vi "Test-Climb.vi"() -> ()   [LabVIEW 2023]
doc: "This VI implements the framework and scheduler for your robotics program. It should not be necessary to modify the framework. You are expected to add your code to the VIs called from Robot Main - the ones located in the Team Code folder within the project."
uses:
  <vilib>/Rock Robotics/WPI/DriverStation/WPI_DriverStationRobotMode2.ctl
  Climb/ClimbStates.ctl
  Robot Global Data.vi
  <vilib>/Rock Robotics/WPI/ThirdParty/JAS_Junk/TrajLib/Trajectory_Library.lvlib
panel:
  out "ClimbStates":T1
  in  "ClimbIncReach":bool
  in  "ClimbIncPull":bool
  in  "ClimbReach":bool
  in  "ClimbPull":bool
  in  "ClimbRest":bool
  out "Wrist Chart":T2(graph)
  out "Battery_Volts":dbl format="%9.1f"
  out "Climbe SP Deg":dbl format="%9.1f"
  out "At Outer Limit":bool
  out "At Inner Limit":bool
  out "Climb Anble Deg":dbl format="%9.1f"
  out "Robot Mode":T3
  out "MotorOutDmd":dbl format="%9.2f"
  in  "error in (no error)":errorcluster
  in  "Finish":bool
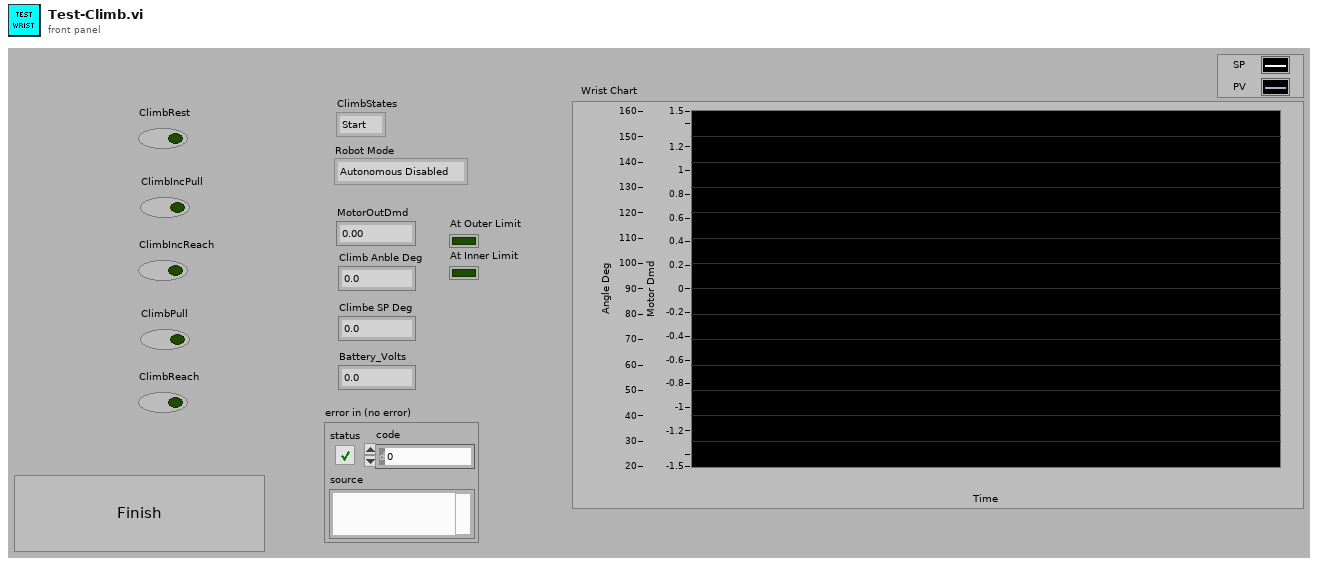
[diagram p1: front panel]
types:
  T1 = typedef "ClimbStates.ctl" = enum16{"Start", "WaitForCommands", "ClimbRest", "ClimbReach", "ClimbPull"}
  T2 = cluster{"ElevatorPosDemandHeight":dbl, "ElevHeightInch":dbl, "MotorDemand":dbl}
  T3 = typedef "WPI_DriverStationRobotMode2.ctl" = enum16{"Autonomous Disabled", "Autonomous Enabled", "Teleop Disabled", "Teleop Enabled", "Disconnected", "Finish", "Test Disabled", "Test Enabled", "Emergency Stopped"}
  T4 = cluster{"WristSP Deg 2":dbl, "ClimbPositionDegrees":dbl, "MotorDemand":dbl}
  T5 = typedef "WPI_DriverStationMatch Info.ctl" = cluster{"Autonomous Elapsed Seconds":dbl, "TeleOp Elapsed Seconds":dbl, "Disabled Elapsed Seconds":dbl, "Visited Autonomous":bool, "Visited TeleOp":bool, "Visited Disabled":bool, "Autonomous Settings":cluster{"Autonomous Style":enum16{"Iterative", "Independent"}, "VI Refnum":refnum<vi>}}
  T6 = typedef "WPI_DriverStationDerivedRobotMode.ctl" = enum16{"Init", "Execute", "Stop"}
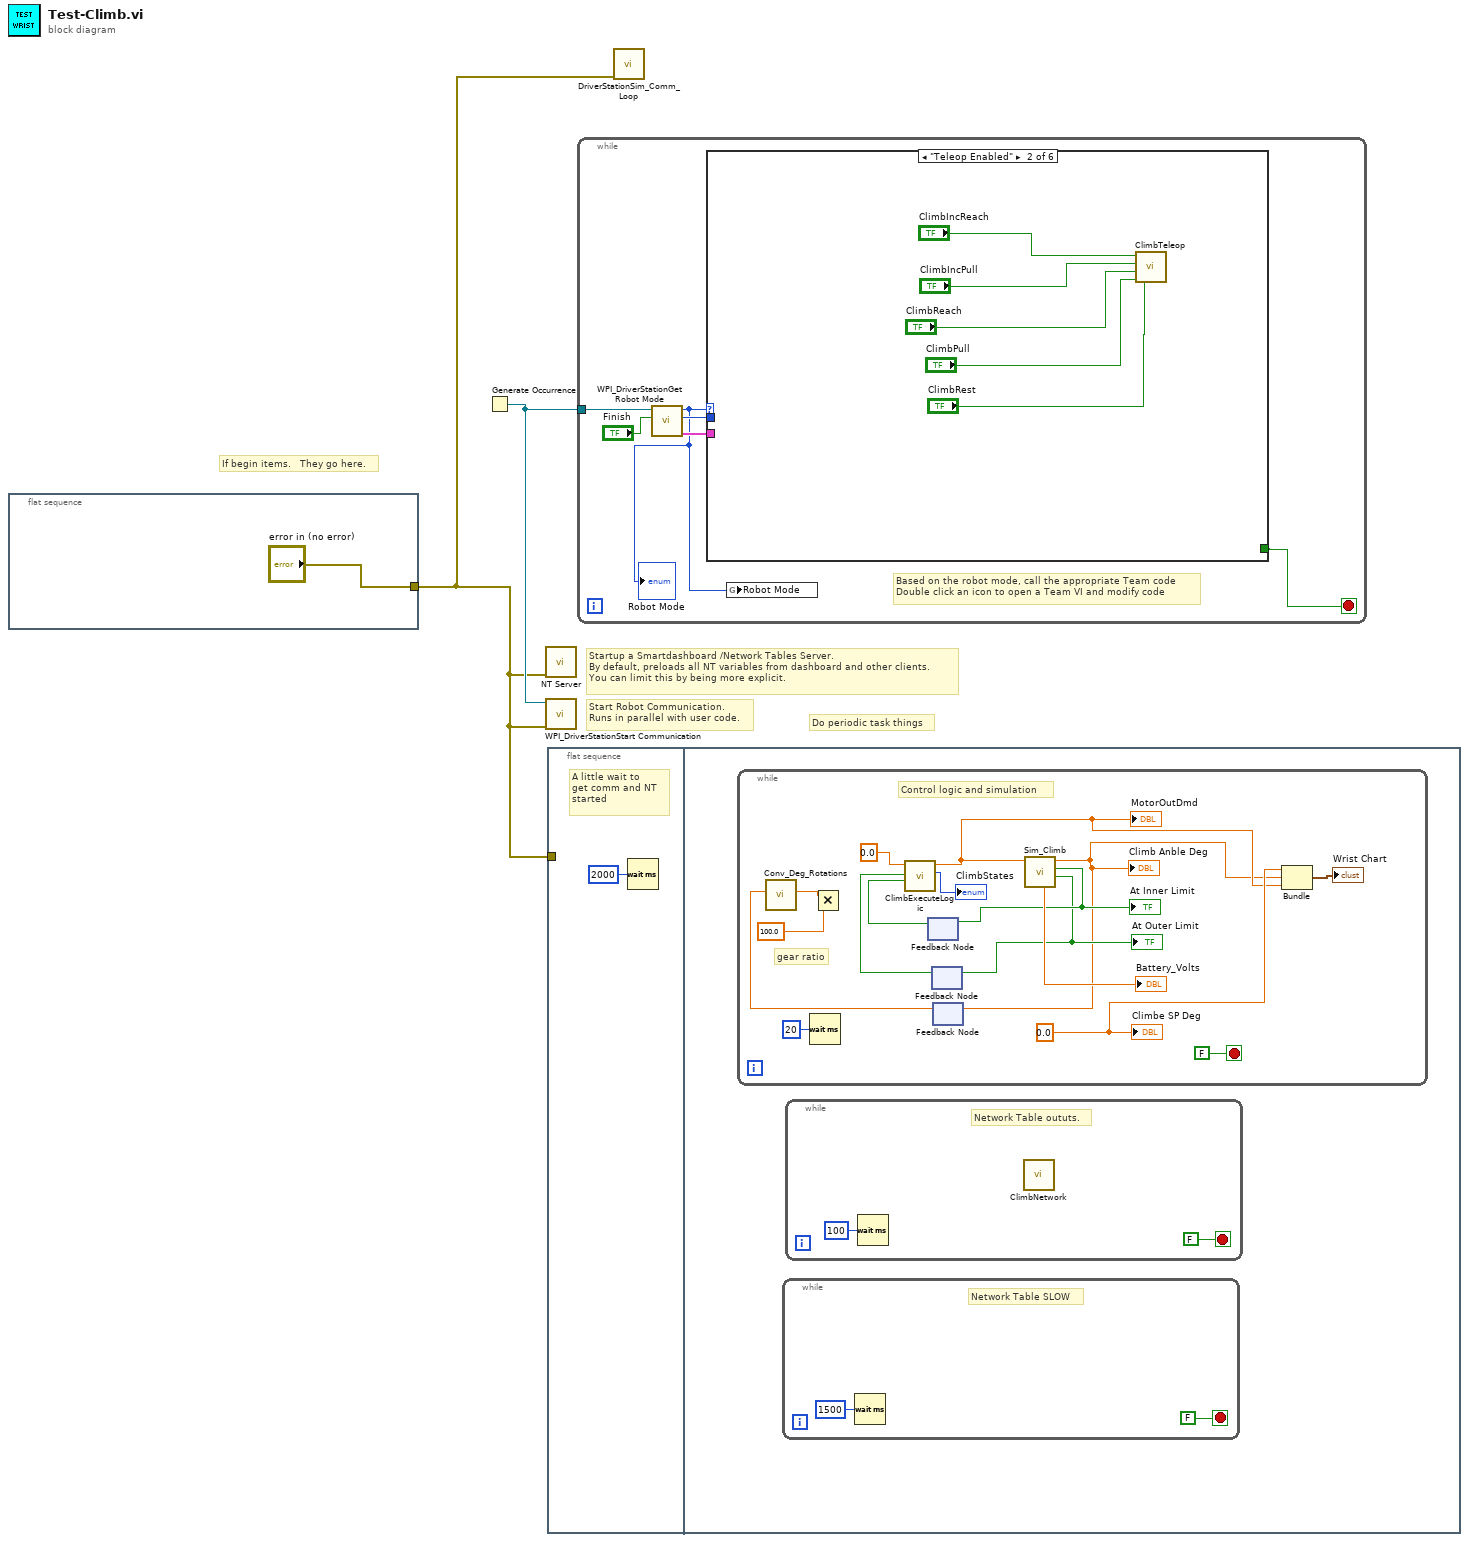
[diagram p0: block diagram]
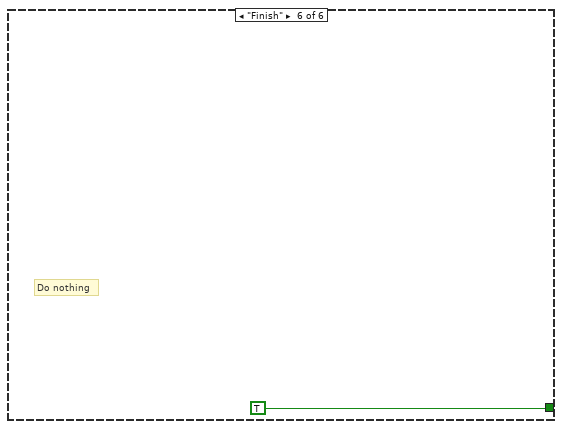
[diagram p6: hidden frame]
diagram:
  # "If begin items.   They go here."
  # "Do periodic task things"
  # "Startup a Smartdashboard /Network Tables Server.\nBy default, preloads all NT variables from dashboard and other clients.\nYou can limit this by being more explicit."
  # "Start Robot Communication.\nRuns in parallel with user code."
  n1 = flat-sequence {
    tunnel: ["error in (no error)"] -> w1
    frame #0 {
    }
  }
  n2 = Generate Occurrence() -> (w2:refnum<k4>)
  n3 = call <vilib>:"NT Server.vi"("error in (no error)"=w1) -> ()  [unwired: 10 in, 1 out]
  n4 = call <vilib>:"WPI_DriverStationStart Communication.vi"("error in (no error)"=w1, "occurrence"=w2) -> ()  [unwired: 1 in, 9 out]
  n5 = flat-sequence {
    tunnel: w1 -> [_]
    frame #0 {
      # "A little wait to\nget comm and NT\nstarted"
      n6 = Wait (ms)(milliseconds to wait=u32 2000) -> ()  [unwired: 1 out]
    }
    frame #1 {
      n7 = while {
        stop <- FALSE stop-if-true
        w20 = 0.0 ("WristSP Deg 2")
        # "gear ratio"
        # "Control logic and simulation"
        n8 = Wait (ms)(milliseconds to wait=u32 20) -> ()  [unwired: 1 out]
        n9 = feedback #1() -> (w11:bool)  [unwired: 1 in]
        n10 = feedback #2() -> (w10:bool)  [unwired: 1 in]
        n11 = call "ClimbExecuteLogic.vi"("Rev"=w11, "Fwd"=w10, "SensorPosition"=0.0) -> ("ClimbStates"=→"ClimbStates":T1, "MotorDemand"=w19:dbl)  [unwired: 6 in, 1 out]
        "MotorOutDmd" <- w19
        n12 = feedback #3() -> (w13:dbl)  [unwired: 1 in]
        n13 = call <vilib>:"Conv_Deg_Rotations.vi"("Degrees"=w13) -> ("Rotations"=w16:dbl)  [unwired: 10 in]
        n14 = Multiply(x=w16, y=100.0) -> ()  [unwired: 1 out]
        n15 = call "Sim_Climb.vi"("Motor1 Dmd"=w19) -> ("At Outer Limit"=w17:bool, "At Climbed Limit"=w18:bool, "ClimbPositionDegrees"=w14:dbl, "Voltage"=→"Battery_Volts":dbl)  [unwired: 6 in, 1 out]
        "Climb Anble Deg" <- w14
        "At Inner Limit" <- w18
        "At Outer Limit" <- w17
        n16 = feedback-in #1(w18) -> ()
        n17 = feedback-in #2(w17) -> ()
        n18 = feedback-in #3(w14) -> ()
        n19 = Bundle("WristSP Deg 2"=w20, "ClimbPositionDegrees"=w14, "MotorDemand"=w19) -> (→"Wrist Chart":T4)  [unwired: 1 in]
        "Climbe SP Deg" <- w20
      }
      n20 = while {
        stop <- FALSE stop-if-true
        # "Network Table SLOW"
        n21 = Wait (ms)(milliseconds to wait=u32 1500) -> ()  [unwired: 1 out]
      }
      n22 = while {
        stop <- FALSE stop-if-true
        # "Network Table oututs."
        n23 = Wait (ms)(milliseconds to wait=u32 100) -> ()  [unwired: 1 out]
        n24 = call "ClimbNetwork.vi"() -> ()  [unwired: 11 in, 1 out]
      }
    }
  }
  n25 = while {
    tunnel: w2 -> [w30]
    stop <- w25 stop-if-true
    # "Based on the robot mode, call the appropriate Team code\nDouble click an icon to open a Team VI and modify code"
    n26 = call <vilib>:"WPI_DriverStationGet Robot Mode.vi"("Finish"="Finish", "DS Occurrence"=w30) -> ("Match Info out"=w27:T5, "Call Context"=w29:T6, "Robot Mode"=w26:T3)  [unwired: 7 out]
    "Robot Mode" <- w26
    n27 = case shown="\"Teleop Enabled\"" w26 {
      tunnel: w29 -> [_ _ _ _ _ _]
      tunnel: w27 -> [_ _ _ _ _ _]
      tunnel: [_ _ _ _ _ TRUE] -> w25
      frame "Autonomous Enabled" {
        # "Do nothing...."
      }
      frame "Teleop Enabled" {
        n28 = call "ClimbTeleop.vi"("ClimbRest"="ClimbRest", "ClimbPull"="ClimbPull", "ClimbReach"="ClimbReach", "ClimbIncPull"="ClimbIncPull", "ClimbIncReach"="ClimbIncReach") -> ()  [unwired: 7 in]
      }
      frame "Test Disabled", "Test Enabled" {
        # "Do nothing"
      }
      frame "Autonomous Disabled", "Teleop Disabled" {
        # "Do nothing."
      }
      frame "Disconnected", Default {
        # "Driver Station packet didn't arrive.\nPossibly useful for diagnostics"
      }
      frame "Finish" {
        # "Do nothing"
      }
    }
    n29 = global write "Robot Global Data.vi" "Robot Mode"(w26) -> ()
  }
  n30 = call <vilib>:"DriverStationSim_Comm_Loop.vi"("error in (no error)"=w1) -> ()  [unwired: 11 in]
